vi "Read Configuration.vi"(8 "error in (no error)":errorcluster, 11 "Error Handler In":refnum<class "Error Handler.lvclass">) -> (0 "error out":errorcluster, 3 "Error Handler Out":refnum<class "Error Handler.lvclass">)   [LabVIEW 2020, in "Error Handler.lvclass"]
doc: "Method that read any necessay configurations from config file or potentially configure hard coded values. The specified configuration file is validated and loaded."
uses:
  Error Handler.lvclass
  Process/Process.lvclass
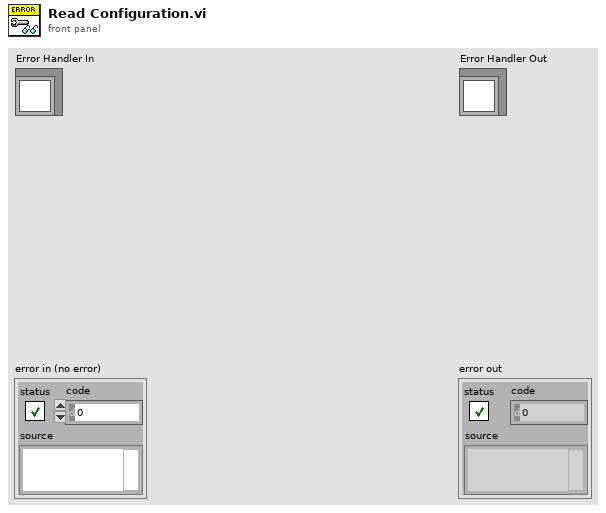
[diagram p1: front panel]
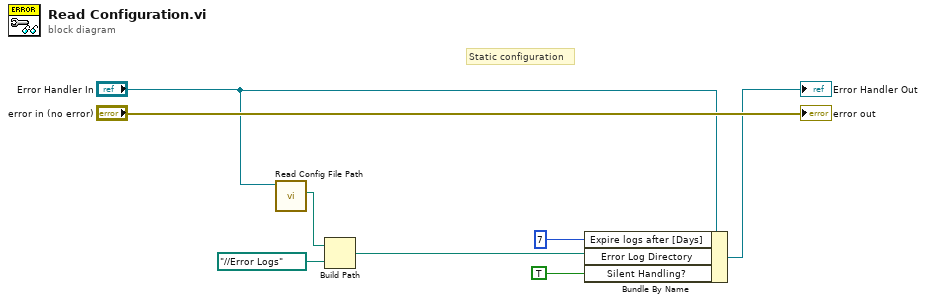
[diagram p0: block diagram]
diagram:
  # "Static configuration"
  n1 = call "Read Config File Path.vi"("Process In"="Error Handler In") -> ("Config File Path"=w1:path)  [unwired: 9 in, 1 out]
  n2 = Build Path(base path=w1, name or relative path=path "../../Error Logs") -> (appended path=w3:path)
  n3 = Bundle By Name(cluster="Error Handler In", "Expire logs after [Days]"=7 ("value"), "Error Log Directory"=w3, "Silent Handling?"=TRUE ("value")) -> (→"Error Handler Out":refnum<class "Error Handler.lvclass">)
  "error out" <- "error in (no error)"
